vi "00-tmp.vi"() -> ()   [LabVIEW 2018]
uses:
  LV-0mq-Julia_roundtrip-lib.lvlib
  Commands.ctl
  Server or client state.ctl
  StackFrame.ctl
  detailed error info.ctl
  jl-scripts path.vi
  ee5840cc-008f-4eed-b97b-e1d8236a7ae0.vi
  placeholder arguments cluster.ctl
  Bindata description.ctl
panel:
  out "binary data received":u8[](array[numeric])
  in  "Bindata & descr in":cluster{"bindata_descr":T1[], "bindata":u8[]}
  in  "Arguments 2":T2
  in  "Arguments 1":T2
  in  "fun2call":string
  in  "next":bool
  out "x+y":dbl=nan
  out "detailed error info":T3
  out "current error":errorcluster
  out "final error":errorcluster
  out "short err code":u8
  in  "stop":bool
  out "ZMQ timeout":bool
  out "Julia script file path":path
  out "temporary script path":path
  out "Jl Server state":T5
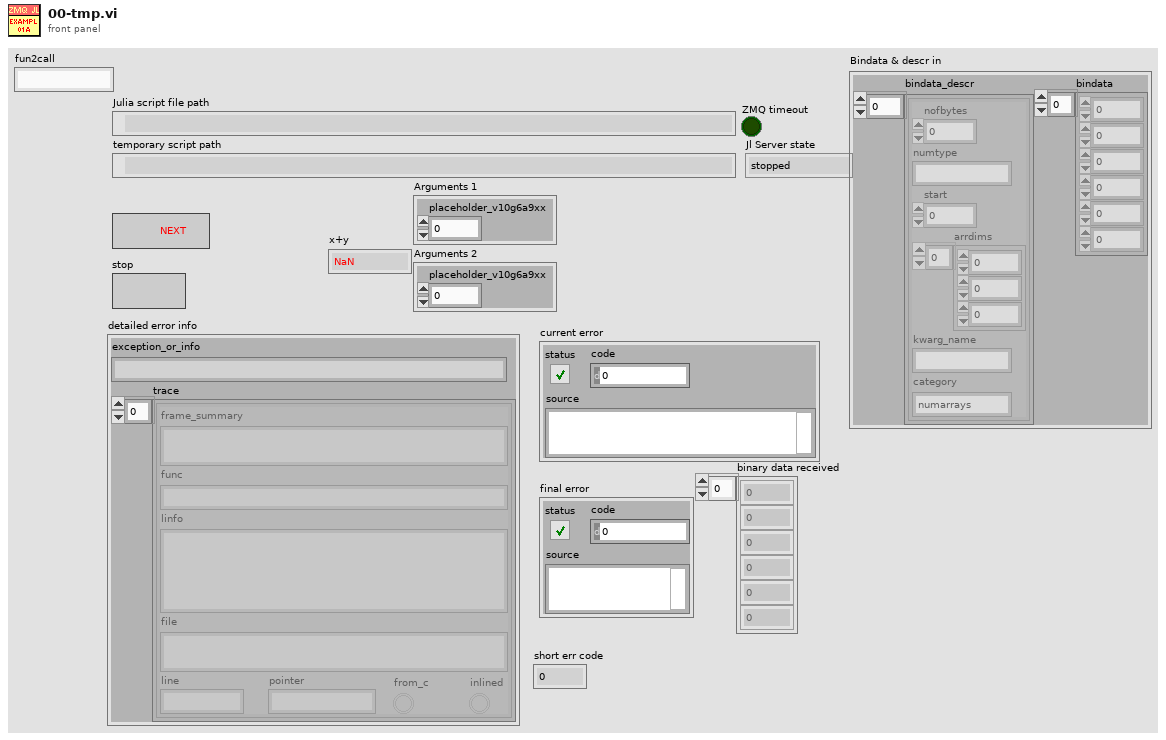
[diagram p1: front panel]
types:
  T1 = typedef "LV-0mq-Julia_roundtrip-lib.lvlib/Bindata description.ctl" = cluster{"nofbytes":i32, "numtype":string, "start":i32, "arrdims":i32[], "kwarg_name":string, "category":string}
  T2 = typedef "LV-0mq-Julia_roundtrip-lib.lvlib/placeholder arguments cluster.ctl" = cluster{"placeholder_v10g6a9xx":i32}
  T3 = typedef "LV-0mq-Julia_roundtrip-lib.lvlib/detailed error info.ctl" = cluster{"exception_or_info":string, "trace":T4[]}
  T4 = typedef "LV-0mq-Julia_roundtrip-lib.lvlib/StackFrame.ctl" = cluster{"frame_summary":string, "func":string, "linfo":string, "file":string, "line":i32, "pointer":u64, "from_c":bool, "inlined":bool}
  T5 = typedef "LV-0mq-Julia_roundtrip-lib.lvlib/Server or client state.ctl" = enum16{"stopped", "running", "unknown"}
  T6 = typedef "LV-0mq-Julia_roundtrip-lib.lvlib/Commands.ctl" = enum16{"Start Jl-server & Init LV-client", "Send request & Get response ", "Stop Jl-server & Cleanup LV-client", "Cleanup LV-client", "Start Jl-server", "Stop Jl-server", "Init LV-Client", "Cleanup LV-Client", "(not allowed)", "Set LV Client state", "Set Jl Server state", "set ZMQ timeout", "read ZMQ timeout", "read-out state"}
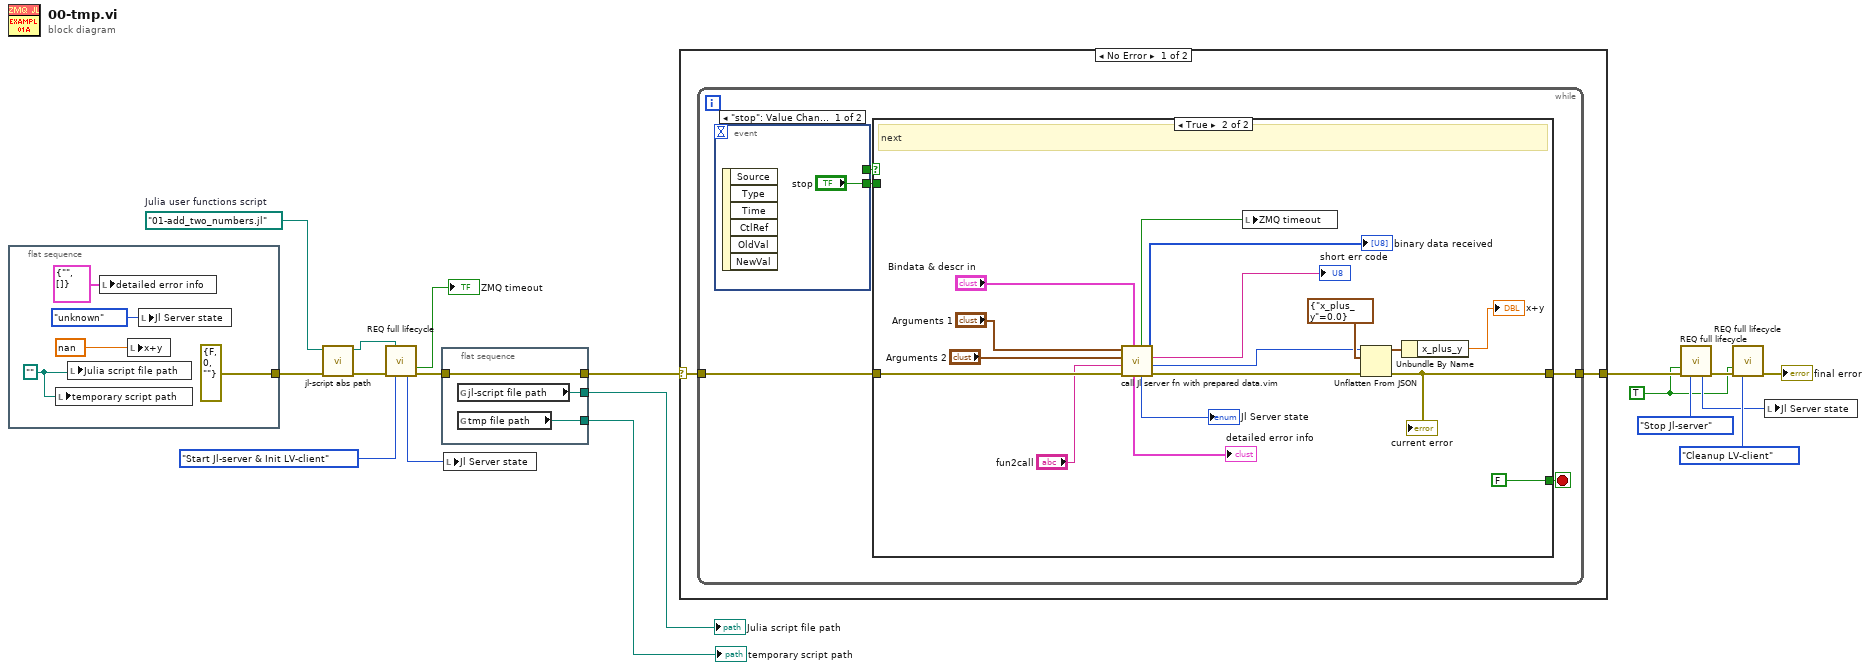
[diagram p0: block diagram]
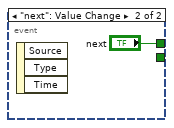
[diagram p2: hidden frame]
diagram:
  w4 = path "01-add_two_numbers.jl"  # Julia user functions script
  w1 = TRUE ("Force command")
  n1 = flat-sequence {
    tunnel: [errorcluster {"status"=FALSE, "code"=0, "source"=""} ("error in (no error)")] -> w2
    frame #0 {
      w19 = path ""
      n2 = local write "temporary script path"(w19) -> ()
      n3 = local write "Julia script file path"(w19) -> ()
      n4 = local write "detailed error info"(T3 {"exception_or_info"="", "trace"=[]} ("detailed error info")) -> ()
      n5 = local write "x+y"(nan ("Server response")) -> ()
      n6 = local write "Jl Server state"(Server_or_client_state."unknown" ("Jl Server state out")) -> ()
    }
  }
  n7 = call "jl-script abs path.vi"("error in (no error)"=w2, "Julia user functions script"=w4) -> ("error out"=w5:errorcluster, "script abs path"=w6:path)  [unwired: 8 in]
  n8 = call "REQ full lifecycle.vi"("Julia user functions script"=w6, "error in"=w5, "command"=Commands."Start Jl-server & Init LV-client") -> ("timeout?"=→"ZMQ timeout":bool, "Jl Server state out"=w8:T5, "error out"=w7:errorcluster)  [unwired: 6 in, 4 out]
  n9 = flat-sequence {
    tunnel: [w26] -> w13
    tunnel: w7 -> [w26]
    tunnel: [w25] -> w11
    tunnel: [w24] -> w12
    frame #0 {
      n10 = global read "jl-scripts path.vi" "jl-script file path"() -> (w25:path)
      n11 = global read "jl-scripts path.vi" "tmp file path"() -> (w24:path)
    }
  }
  n12 = local write "Jl Server state"(w8) -> ()
  n13 = case shown="No Error" w13 {
    selector: w13 -> [w27 w55]
    tunnel: [w28 w55] -> w18
    frame No Error {
      n14 = while {
        tunnel: w27 -> [w32]
        tunnel: [w33] -> w28
        stop <- w30 stop-if-true
        n15 = event shown="[0] \"stop\": Value Change" {
          selector: _ -> [_ _]
          dyn-events: _ -> [_ _]
          timeout: _ -> [_ _]
          tunnel: [_ "next"] -> w31
          tunnel: ["stop" _] -> w29
          event "stop": Value Change {
            n16 = event-data() -> ()  [unwired: 1 in, 6 out]
          }
          event "next": Value Change {
            n17 = event-data() -> ()  [unwired: 1 in, 3 out]
          }
        }
        n18 = case shown="True" w31 {
          tunnel: [w37 w50] -> w33
          tunnel: w32 -> [w37 w52]
          tunnel: [w36 FALSE ("stop this VI only")] -> w30
          tunnel: w29 -> [w36 _]
          frame False {
            # "stop"
          }
          frame True {
            # "next"
            n19 = call "call Jl server fn with prepared data.vim"("Bindata & descr in"="Bindata & descr in", "error in (no error)"=w52, "fun2call"="fun2call", "Arguments in"="Arguments 2", "Arguments 1"="Arguments 1") -> ("error out"=w44:errorcluster, "Jl Server state out"=w46:T5, "JSON received"=→"short err code":string, "binary data received"=→"binary data received":u8[], "return code"=→"Jl Server state":u8, "timeout?"=w43:bool, "detailed error info"=→"detailed error info":T3)
            n20 = local write "ZMQ timeout"(w43) -> ()
            n21 = Unflatten From JSON(JSON string=w46, type and defaults=cluster{"x_plus_y":dbl} {"x_plus_y"=0.0} ("parsed response"), error in (no error)=w44) -> (value=w53:cluster{"x_plus_y":dbl}, error out=w50:errorcluster)  [unwired: 4 in]
            "current error" <- w50
            n22 = Unbundle By Name(w53) -> ("x_plus_y"=→"x+y":dbl)
          }
        }
      }
    }
    frame Error {
    }
  }
  n23 = call "REQ full lifecycle.vi"("Force command"=w1, "error in"=w18, "command"=Commands."Stop Jl-server") -> ("Jl Server state out"=w10:T5, "error out"=w16:errorcluster)  [unwired: 6 in, 5 out]
  n24 = call "REQ full lifecycle.vi"("Force command"=w1, "error in"=w16, "command"=Commands."Cleanup LV-client") -> ("error out"=→"final error":errorcluster)  [unwired: 6 in, 6 out]
  n25 = local write "Jl Server state"(w10) -> ()
  "temporary script path" <- w12
  "Julia script file path" <- w11
